vi "Start Flow (Continuous).vi"(6 "Reset Volume Counter (T)":bool=TRUE, 7 "Pump ID (0:A)":T2, 8 "error in (no error)":errorcluster, 9 "Direction (0:Aspirate)":T1, 11 "VISA resource in":refnum<visa-resource-name>) -> (0 "error out":errorcluster, 3 "VISA resource out":refnum<visa-resource-name>)   [LabVIEW 2020, in "Global FIA milliGAT.lvlib"]
doc: "Starts the pump flowing continuously."
uses:
  <instrlib>/RxnRover/Global FIA milliGAT 3.14/Global FIA milliGAT.lvlib
  <instrlib>/RxnRover/Global FIA milliGAT 3.14/Public/Utility/Pump Address.ctl
  <instrlib>/RxnRover/Global FIA milliGAT 3.14/Public/Utility/Pump Direction.ctl
  <instrlib>/RxnRover/Global FIA milliGAT 3.14/Private/Pump Parameter.ctl
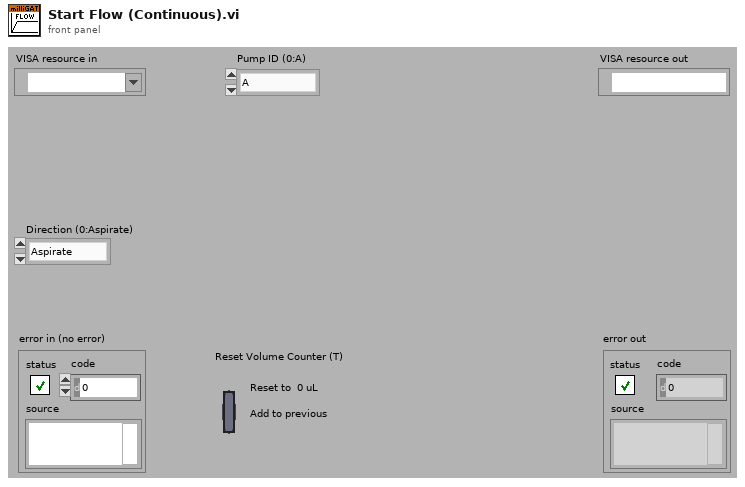
[diagram p1: front panel]
types:
  T1 = typedef "Global FIA milliGAT.lvlib/Pump Direction.ctl" = enum16{"Aspirate", "Dispense"}
  T2 = typedef "Global FIA milliGAT.lvlib/Pump Address.ctl" = enum16{"A", "B", "C", "D", "E", "F", "G", "H", "I", "J", "K", "L", "M", "N", "O", "P", "Q", "R", "S", "T", "U", "V", "W", "X", "Y", "Z", "a", "b", "c", "d", "e", "f", "g", "h", "i", "j", "k", "l", "m", "n", "o", "p", "q", "r", "s", "t", "u", "v", "w", "x", "y", "z", "0", "1", "2", "3", "4", "5", "6", "7", "8", "9"}
  T3 = typedef "Global FIA milliGAT.lvlib/Pump Parameter.ctl" = enum16{"Enabled", "EU", "EU Calibration Factor", "Fixed Asp or Disp", "Starting Position", "Starting Flow", "Peak Flow", "Flow Acceleration", "Flow Deceleration", "Session Volume", "Max Pressure", "Backlash (usteps)", "BL Calibration Factor", "BL Correction Enabled", "Min Flow", "Max Flow", "Min Acceleration", "Max Acceleration", "Service Volume", "Life Volume"}
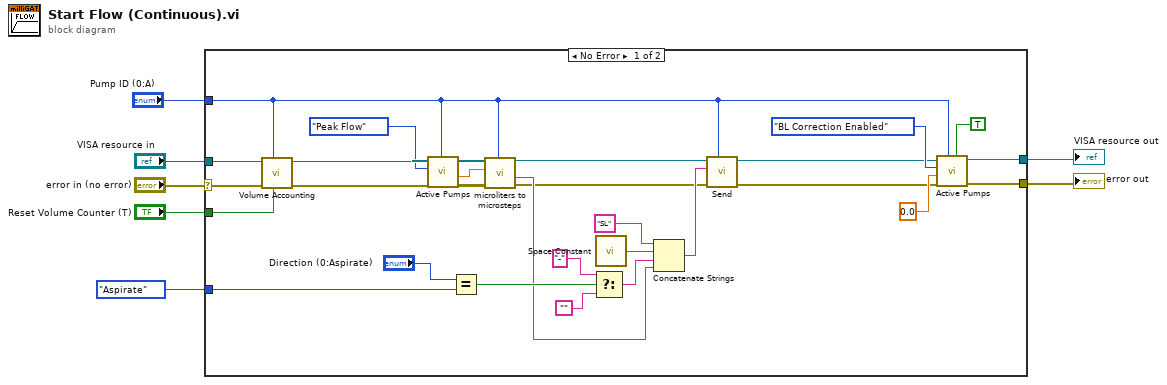
[diagram p0: block diagram]
diagram:
  n1 = case shown="No Error" "error in (no error)" {
    selector: "error in (no error)" -> [w8 w37]
    tunnel: Pump_Direction."Aspirate" ("y") -> [w33 _]
    tunnel: "VISA resource in" -> [w27 w38]
    tunnel: "Reset Volume Counter (T)" -> [w26 _]
    tunnel: [w11 w38] -> w4
    tunnel: [w10 w37] -> w3
    tunnel: "Pump ID (0:A)" -> [w9 _]
    frame No Error {
      n2 = call <instrlib>:"Volume Accounting.vi"("Reset Volume Counter (T)"=w26, "Pump ID (0:A)"=w9, "error in (no error)"=w8, "VISA resource in"=w27) -> ("error out"=w14:errorcluster, "VISA resource out"=w15:refnum<visa-resource-name>)  [unwired: 6 in]
      n3 = call <instrlib>:"Active Pumps.vi"("Pump ID (0:A)"=w9, "error in (no error)"=w14, "Parameter"=Pump_Parameter."Peak Flow", "VISA resource in"=w15) -> ("error out"=w20:errorcluster, "Value out"=w18:dbl, "VISA resource out"=w21:refnum<visa-resource-name>)  [unwired: 4 in, 1 out]
      n4 = Equal?(x="Direction (0:Aspirate)", y=w33) -> (x = y?=w28:bool)
      n5 = call <instrlib>:"microliters to microsteps.vi"("Pump ID (0:A)"=w9, "error in (no error)"=w20, "Microliters (0)"=w18, "VISA resource in"=w21) -> ("error out"=w22:errorcluster, "Microsteps (STR)"=w23:string, "VISA resource out"=w24:refnum<visa-resource-name>)  [unwired: 4 in, 1 out]
      n6 = Select(t="-", s=w28, f="") -> (s? t:f=w30:string)
      n7 = call <vilib>:"Space Constant.vi"() -> ("String"=w35:string)
      n8 = Concatenate Strings("SL", w35, w30, w23) -> (w29:string)
      n9 = call <instrlib>:"Send.vi"("Pump ID (0:A)"=w9, "error in (no error)"=w22, "Command"=w29, "VISA resource in"=w24) -> ("error out"=w12:errorcluster, "VISA resource out"=w13:refnum<visa-resource-name>)  [unwired: 5 in, 1 out]
      n10 = call <instrlib>:"Active Pumps.vi"("Action (F:Read)"=TRUE, "Pump ID (0:A)"=w9, "error in (no error)"=w12, "Value in"=0.0, "Parameter"=Pump_Parameter."BL Correction Enabled", "VISA resource in"=w13) -> ("error out"=w10:errorcluster, "VISA resource out"=w11:refnum<visa-resource-name>)  [unwired: 2 in, 2 out]
    }
    frame Error {
    }
  }
  "VISA resource out" <- w4
  "error out" <- w3
